vi "Global_2.vi"() -> ()   [LabVIEW 2016]
panel:
  in  "Stop Button_2":bool
  out "Numeric Control_2":dbl
  out "Boolean_2":bool
  out "Comunicacion_2":string
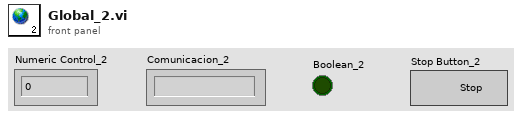
[diagram p1: front panel]
diagram:
